vi "input.vi"(8 "error in":errorcluster, 10 "data table in":T1, 11 "Engine to Engine Communication runtime in":refnum<class "E2E Runtime (RT FIFO).lvclass">) -> (0 "error out":errorcluster, 2 "data table out":T1, 3 "Engine to Engine Communication runtime out":refnum<class "E2E Runtime (RT FIFO).lvclass">)   [LabVIEW 2015, in "E2E Runtime (RT FIFO).lvclass"]
doc: "Provides an interface for reading data from a module at runtime. While this interface performs no operations, a child should provide an override which may read from any open sessions, references, or interfaces."
uses:
  E2E Runtime (RT FIFO).lvclass
  <vilib>/NI/Tag Bus/table/data table.ctl
  E2E Runtime (RT FIFO).lvclass/E2E Runtime (RT FIFO).ctl
  <vilib>/NI/Tag Bus/table/data polymorphs/write all/write all Doubles.vi
  <vilib>/NI/Tag Bus/table/data polymorphs/write all/write all Singles.vi
  <vilib>/NI/Tag Bus/table/data polymorphs/write all/write all I64s.vi
  <vilib>/NI/Tag Bus/table/data polymorphs/write all/write all I32s.vi
  <vilib>/NI/Tag Bus/table/data polymorphs/write all/write all I16s.vi
  <vilib>/NI/Tag Bus/table/data polymorphs/write all/write all I8s.vi
  <vilib>/NI/Tag Bus/table/data polymorphs/write all/write all U64s.vi
  <vilib>/NI/Tag Bus/table/data polymorphs/write all/write all U32s.vi
  <vilib>/NI/Tag Bus/table/data polymorphs/write all/write all U16s.vi
  <vilib>/NI/Tag Bus/table/data polymorphs/write all/write all U8s.vi
  <vilib>/NI/Tag Bus/table/data polymorphs/write all/write all Booleans.vi
  <vilib>/NI/Tag Bus/tag bus error generator.vi
  <vilib>/NI/Tag Bus/table/data table.lvlib
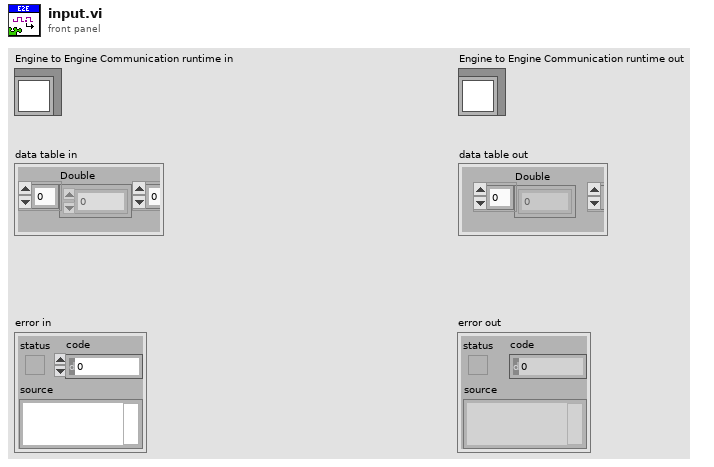
[diagram p1: front panel]
types:
  T1 = typedef "tag bus.lvlib/data table.lvlib/data table.ctl" = cluster{"Double":dbl[], "Single":sgl[], "I64":i64[], "I32":i32[], "I16":i16[], "I8":i8[], "U64":u64[], "U32":u32[], "U16":u16[], "U8":u8[], "Boolean":bool[], "String":string[], "Array of Double":cluster{"DBL Array":dbl[]}[], "Array of Single":cluster{"SGL Array":sgl[]}[], "Array of I64":cluster{"I64 Array":i64[]}[], "Array of I32":cluster{"I32 Array":i32[]}[], "Array of I16":cluster{"I16 Array":i16[]}[], "Array of I8":cluster{"I8 Array":i8[]}[], "Array of U64":cluster{"U64 Array":u64[]}[], "Array of U32":cluster{"U32 Array":u32[]}[], "Array of U16":cluster{"U16 Array":u16[]}[], "Array of U8":cluster{"U8 Array":u8[]}[], "Array of Boolean":cluster{"Boolean Array":bool[]}[], "Array of String":cluster{"String Array":string[]}[]}
  T2 = typedef "tag bus.lvlib/tag descriptor.lvclass/Data Type.ctl" = enum16{"Double", "Single", "I64", "I32", "I16", "I8", "U64", "U32", "U16", "U8", "Boolean", "String", "Array of Double", "Array of Single", "Array of I64", "Array of I32", "Array of I16", "Array of I8", "Array of U64", "Array of U32", "Array of U16", "Array of U8", "Array of Boolean", "Array of String"}
  T3 = typedef "E2E Runtime (RT FIFO).lvclass/Data FIFOs.ctl" = cluster{"Double":refnum<k33>, "Single":refnum<k33>, "I64":refnum<k33>, "I32":refnum<k33>, "I16":refnum<k33>, "I8":refnum<k33>, "U64":refnum<k33>, "U32":refnum<k33>, "U16":refnum<k33>, "U8":refnum<k33>, "Boolean":refnum<k33>}
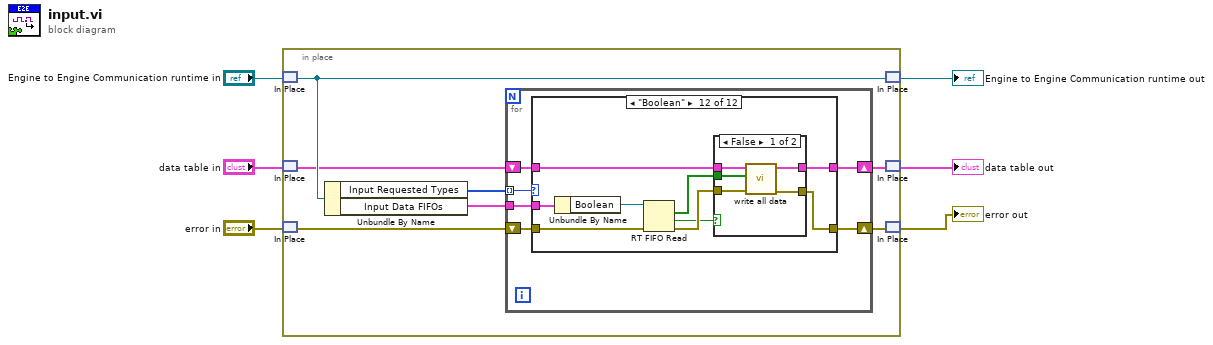
[diagram p0: block diagram]
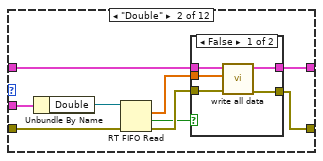
[diagram p3: hidden frame]
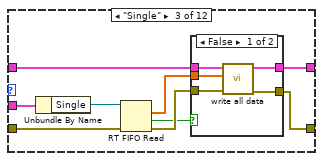
[diagram p5: hidden frame]
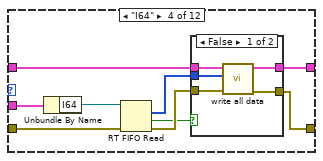
[diagram p7: hidden frame]
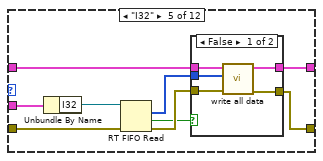
[diagram p9: hidden frame]
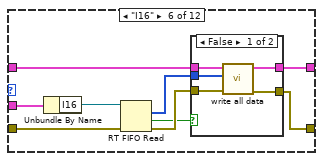
[diagram p11: hidden frame]
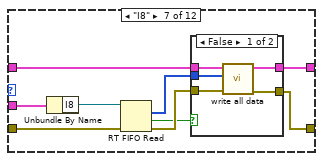
[diagram p13: hidden frame]
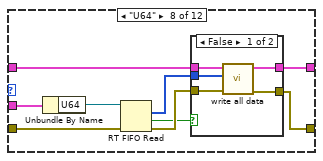
[diagram p15: hidden frame]
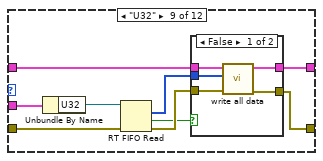
[diagram p17: hidden frame]
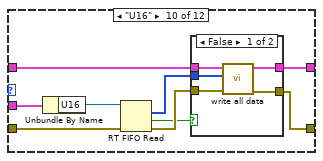
[diagram p19: hidden frame]
diagram:
  n1 = in-place {
    n2 = in-place-match #1("Engine to Engine Communication runtime in") -> (w13:refnum<class "E2E Runtime (RT FIFO).lvclass">)
    n3 = in-place-match #2("data table in") -> (w12:T1)
    n4 = in-place-match #3("error in") -> (w9:errorcluster)
    n5 = Unbundle By Name(w13) -> ("Input Requested Types"=w11:T2[], "Input Data FIFOs"=w10:T3)
    n6 = for {
      tunnel: w11 -> [w19] mode=indexing
      tunnel: w10 -> [w18]
      shift-right: [w15] -> w7
      shift-left: w9 -> [w17]
      shift-right: [w14] -> w8
      shift-left: w12 -> [w16]
      n7 = case shown="\"Boolean\"" w19 {
        tunnel: w18 -> [_ w28 w44 w60 w76 w92 w108 w124 w140 w156 w172 w188]
        tunnel: w17 -> [w21 w29 w45 w61 w77 w93 w109 w125 w141 w157 w173 w189]
        tunnel: w16 -> [w20 w27 w43 w59 w75 w91 w107 w123 w139 w155 w171 w187]
        tunnel: [w21 w24 w40 w56 w72 w88 w104 w120 w136 w152 w168 w184] -> w15
        tunnel: [w20 w23 w39 w55 w71 w87 w103 w119 w135 w151 w167 w183] -> w14
        frame Default {
        }
        frame "Double" {
          n8 = Unbundle By Name(w28) -> ("Double"=w30:refnum<k33>)
          n9 = RT FIFO Read(0:w30, 3:w29) -> (9:w26:dbl[], 10:w22:bool, 11:w25:errorcluster)  [unwired: 2 in, 2 out]
          n10 = case shown="False" w22 {
            tunnel: w27 -> [w35 w37]
            tunnel: w26 -> [w34 _]
            tunnel: w25 -> [w33 w36]
            tunnel: [w32 w36] -> w24
            tunnel: [w31 w37] -> w23
            frame False {
              n11 = call-poly <vilib>:"write all data.vi"("error in"=w33, "values"=w34, "data table in"=w35) -> ("error out"=w32:errorcluster, "data table out"=w31:T1)  [unwired: 7 in]
            }
            frame True {
            }
          }
        }
        frame "Single" {
          n12 = Unbundle By Name(w44) -> ("Single"=w46:refnum<k33>)
          n13 = RT FIFO Read(0:w46, 3:w45) -> (9:w42:sgl[], 10:w38:bool, 11:w41:errorcluster)  [unwired: 2 in, 2 out]
          n14 = case shown="False" w38 {
            tunnel: w43 -> [w51 w53]
            tunnel: w42 -> [w50 _]
            tunnel: w41 -> [w49 w52]
            tunnel: [w48 w52] -> w40
            tunnel: [w47 w53] -> w39
            frame False {
              n15 = call-poly <vilib>:"write all data.vi"("error in"=w49, "values"=w50, "data table in"=w51) -> ("error out"=w48:errorcluster, "data table out"=w47:T1)  [unwired: 7 in]
            }
            frame True {
            }
          }
        }
        frame "I64" {
          n16 = Unbundle By Name(w60) -> ("I64"=w62:refnum<k33>)
          n17 = RT FIFO Read(0:w62, 3:w61) -> (9:w58:i64[], 10:w54:bool, 11:w57:errorcluster)  [unwired: 2 in, 2 out]
          n18 = case shown="False" w54 {
            tunnel: w59 -> [w67 w69]
            tunnel: w58 -> [w66 _]
            tunnel: w57 -> [w65 w68]
            tunnel: [w64 w68] -> w56
            tunnel: [w63 w69] -> w55
            frame False {
              n19 = call-poly <vilib>:"write all data.vi"("error in"=w65, "values"=w66, "data table in"=w67) -> ("error out"=w64:errorcluster, "data table out"=w63:T1)  [unwired: 7 in]
            }
            frame True {
            }
          }
        }
        frame "I32" {
          n20 = Unbundle By Name(w76) -> ("I32"=w78:refnum<k33>)
          n21 = RT FIFO Read(0:w78, 3:w77) -> (9:w74:i32[], 10:w70:bool, 11:w73:errorcluster)  [unwired: 2 in, 2 out]
          n22 = case shown="False" w70 {
            tunnel: w75 -> [w83 w85]
            tunnel: w74 -> [w82 _]
            tunnel: w73 -> [w81 w84]
            tunnel: [w80 w84] -> w72
            tunnel: [w79 w85] -> w71
            frame False {
              n23 = call-poly <vilib>:"write all data.vi"("error in"=w81, "values"=w82, "data table in"=w83) -> ("error out"=w80:errorcluster, "data table out"=w79:T1)  [unwired: 7 in]
            }
            frame True {
            }
          }
        }
        frame "I16" {
          n24 = Unbundle By Name(w92) -> ("I16"=w94:refnum<k33>)
          n25 = RT FIFO Read(0:w94, 3:w93) -> (9:w90:i16[], 10:w86:bool, 11:w89:errorcluster)  [unwired: 2 in, 2 out]
          n26 = case shown="False" w86 {
            tunnel: w91 -> [w99 w101]
            tunnel: w90 -> [w98 _]
            tunnel: w89 -> [w97 w100]
            tunnel: [w96 w100] -> w88
            tunnel: [w95 w101] -> w87
            frame False {
              n27 = call-poly <vilib>:"write all data.vi"("error in"=w97, "values"=w98, "data table in"=w99) -> ("error out"=w96:errorcluster, "data table out"=w95:T1)  [unwired: 7 in]
            }
            frame True {
            }
          }
        }
        frame "I8" {
          n28 = Unbundle By Name(w108) -> ("I8"=w110:refnum<k33>)
          n29 = RT FIFO Read(0:w110, 3:w109) -> (9:w106:i8[], 10:w102:bool, 11:w105:errorcluster)  [unwired: 2 in, 2 out]
          n30 = case shown="False" w102 {
            tunnel: w107 -> [w115 w117]
            tunnel: w106 -> [w114 _]
            tunnel: w105 -> [w113 w116]
            tunnel: [w112 w116] -> w104
            tunnel: [w111 w117] -> w103
            frame False {
              n31 = call-poly <vilib>:"write all data.vi"("error in"=w113, "values"=w114, "data table in"=w115) -> ("error out"=w112:errorcluster, "data table out"=w111:T1)  [unwired: 7 in]
            }
            frame True {
            }
          }
        }
        frame "U64" {
          n32 = Unbundle By Name(w124) -> ("U64"=w126:refnum<k33>)
          n33 = RT FIFO Read(0:w126, 3:w125) -> (9:w122:u64[], 10:w118:bool, 11:w121:errorcluster)  [unwired: 2 in, 2 out]
          n34 = case shown="False" w118 {
            tunnel: w123 -> [w131 w133]
            tunnel: w122 -> [w130 _]
            tunnel: w121 -> [w129 w132]
            tunnel: [w128 w132] -> w120
            tunnel: [w127 w133] -> w119
            frame False {
              n35 = call-poly <vilib>:"write all data.vi"("error in"=w129, "values"=w130, "data table in"=w131) -> ("error out"=w128:errorcluster, "data table out"=w127:T1)  [unwired: 7 in]
            }
            frame True {
            }
          }
        }
        frame "U32" {
          n36 = Unbundle By Name(w140) -> ("U32"=w142:refnum<k33>)
          n37 = RT FIFO Read(0:w142, 3:w141) -> (9:w138:u32[], 10:w134:bool, 11:w137:errorcluster)  [unwired: 2 in, 2 out]
          n38 = case shown="False" w134 {
            tunnel: w139 -> [w147 w149]
            tunnel: w138 -> [w146 _]
            tunnel: w137 -> [w145 w148]
            tunnel: [w144 w148] -> w136
            tunnel: [w143 w149] -> w135
            frame False {
              n39 = call-poly <vilib>:"write all data.vi"("error in"=w145, "values"=w146, "data table in"=w147) -> ("error out"=w144:errorcluster, "data table out"=w143:T1)  [unwired: 7 in]
            }
            frame True {
            }
          }
        }
        frame "U16" {
          n40 = Unbundle By Name(w156) -> ("U16"=w158:refnum<k33>)
          n41 = RT FIFO Read(0:w158, 3:w157) -> (9:w154:u16[], 10:w150:bool, 11:w153:errorcluster)  [unwired: 2 in, 2 out]
          n42 = case shown="False" w150 {
            tunnel: w155 -> [w163 w165]
            tunnel: w154 -> [w162 _]
            tunnel: w153 -> [w161 w164]
            tunnel: [w160 w164] -> w152
            tunnel: [w159 w165] -> w151
            frame False {
              n43 = call-poly <vilib>:"write all data.vi"("error in"=w161, "values"=w162, "data table in"=w163) -> ("error out"=w160:errorcluster, "data table out"=w159:T1)  [unwired: 7 in]
            }
            frame True {
            }
          }
        }
        frame "U8" {
          n44 = Unbundle By Name(w172) -> ("U8"=w174:refnum<k33>)
          n45 = RT FIFO Read(0:w174, 3:w173) -> (9:w170:u8[], 10:w166:bool, 11:w169:errorcluster)  [unwired: 2 in, 2 out]
          n46 = case shown="False" w166 {
            tunnel: w171 -> [w179 w181]
            tunnel: w170 -> [w178 _]
            tunnel: w169 -> [w177 w180]
            tunnel: [w176 w180] -> w168
            tunnel: [w175 w181] -> w167
            frame False {
              n47 = call-poly <vilib>:"write all data.vi"("error in"=w177, "values"=w178, "data table in"=w179) -> ("error out"=w176:errorcluster, "data table out"=w175:T1)  [unwired: 7 in]
            }
            frame True {
            }
          }
        }
        frame "Boolean" {
          n48 = Unbundle By Name(w188) -> ("Boolean"=w190:refnum<k33>)
          n49 = RT FIFO Read(0:w190, 3:w189) -> (9:w186:bool[], 10:w182:bool, 11:w185:errorcluster)  [unwired: 2 in, 2 out]
          n50 = case shown="False" w182 {
            tunnel: w187 -> [w195 w197]
            tunnel: w186 -> [w194 _]
            tunnel: w185 -> [w193 w196]
            tunnel: [w192 w196] -> w184
            tunnel: [w191 w197] -> w183
            frame False {
              n51 = call-poly <vilib>:"write all data.vi"("error in"=w193, "values"=w194, "data table in"=w195) -> ("error out"=w192:errorcluster, "data table out"=w191:T1)  [unwired: 7 in]
            }
            frame True {
            }
          }
        }
      }
    }
    n52 = in-place-match #1(w13) -> (→"Engine to Engine Communication runtime out":refnum<class "E2E Runtime (RT FIFO).lvclass">)
    n53 = in-place-match #2(w8) -> (→"data table out":T1)
    n54 = in-place-match #3(w7) -> (→"error out":errorcluster)
  }
